vi "Single Pulse Width.vi"(2 "wfm":dbl[](array[numeric]), 3 "wfm info":T1 {"reserved2" format="%.2f"; "reserved1" format="%.2f"; "offset" format="%^.3e"; "gain" format="%^.3e"; "xIncrement" format="%^.3e"; "relativeInitialX" format="%^.3e"; "absoluteInitialX" format="%^.3e"}) -> (0 "Pulse Width":dbl)   [LabVIEW 2009]
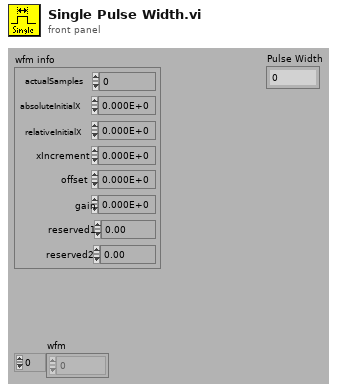
[diagram p1: front panel]
types:
  T1 = cluster{"actualSamples":i32, "absoluteInitialX":dbl, "relativeInitialX":dbl, "xIncrement":dbl, "offset":dbl, "gain":dbl, "reserved1":dbl, "reserved2":dbl}
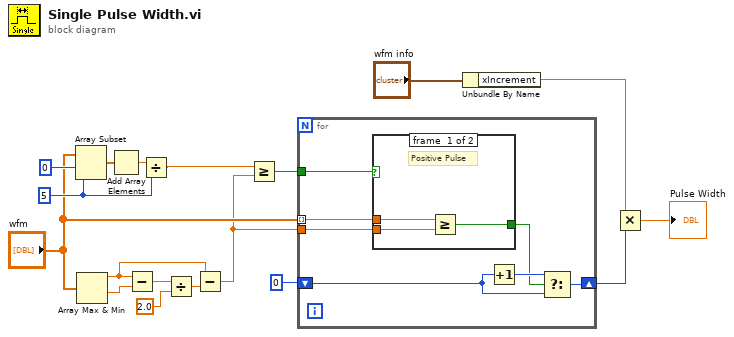
[diagram p0: block diagram]
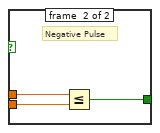
[diagram p2: hidden frame]
diagram:
  w7 = 5 ("length")
  n1 = Array Subset(array="wfm", index=0, length=w7) -> (w9:dbl[])
  n2 = Array Max & Min(array="wfm") -> (max value=w13:dbl, min value=w17:dbl)  [unwired: 2 out]
  n3 = Add Array Elements(numeric array=w9) -> (sum=w8:dbl)
  n4 = Subtract(x=w13, y=w17) -> (x-y=w14:dbl)
  n5 = Divide(x=w8, y=w7) -> (x/y=w5:dbl)
  n6 = Divide(x=w14, y=2.0) -> (x/y=w15:dbl)
  n7 = Subtract(x=w13, y=w15) -> (x-y=w1:dbl)
  n8 = Greater Or Equal?(x=w5, y=w1) -> (x >= y?=w6:bool)
  n9 = for {
    tunnel: w6 -> [w25]
    tunnel: "wfm" -> [w24] mode=indexing
    tunnel: w1 -> [w23]
    shift-right: [w22] -> w2
    shift-left: 0 ("index") -> [w20]
    n10 = case shown="True" w25 {
      tunnel: w24 -> [w27 w31]
      tunnel: w23 -> [w26 w30]
      tunnel: [w28 w29] -> w19
      frame #0 {
        # "Positive Pulse"
        n11 = Greater Or Equal?(x=w27, y=w26) -> (x >= y?=w28:bool)
      }
      frame #1 {
        # "Negative Pulse"
        n12 = Less Or Equal?(x=w31, y=w30) -> (x <= y?=w29:bool)
      }
    }
    n13 = Increment(x=w20) -> (x+1=w21:i32)
    n14 = Select(t=w21, s=w19, f=w20) -> (s? t:f=w22:i32)
  }
  n15 = Unbundle By Name("wfm info") -> ("xIncrement"=w12:dbl)
  n16 = Multiply(x=w12, y=w2) -> (x*y=→"Pulse Width":dbl)
